vi "stm_GetIDfromName_.vi"(9 "Name":string, 11 "MetaData":T1[](array[typedef])) -> (1 "Found":bool, 3 "Meta ID":u16)   [LabVIEW 2013, in "Diagnostics Addon Engine.lvlib"]
doc: "This VI looks up the Meta data index using the Meta data name."
uses:
  Diagnostics Addon Engine.lvlib
  stm_MetaDataElement.ctl
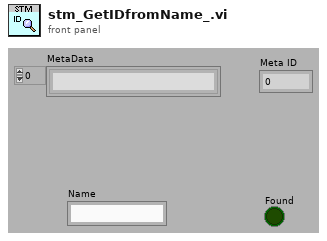
[diagram p1: front panel]
types:
  T1 = typedef "Diagnostics Addon Engine.lvlib/stm_MetaDataElement.ctl" = string
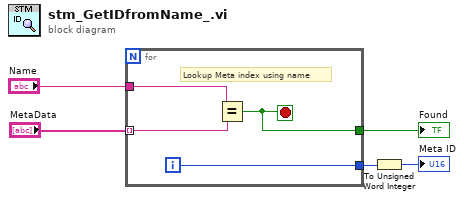
[diagram p0: block diagram]
diagram:
  n1 = for {
    tunnel: "MetaData" -> [w7] mode=indexing
    tunnel: "Name" -> [w9]
    tunnel: [w8] -> w3
    tunnel: [w6] -> w1
    i -> [w8]
    stop <- w6 stop-if-true
    # "Lookup Meta index using name"
    n2 = Equal?(x=w9, y=w7) -> (x = y?=w6:bool)
  }
  "Found" <- w1
  n3 = To Unsigned Word Integer(number=w3) -> (unsigned 16bit integer=→"Meta ID":u16)
